vi "Get Keys.vi"(8 "error in":errorcluster, 11 "Object Entry in":refnum<class "Section.lvclass">) -> (0 "error out":errorcluster, 2 "Keys":refnum<class "Key Name.lvclass">[](array[class]), 3 "Object Entry out":refnum<class "Section.lvclass">)   [LabVIEW 2019, in "Electronic Datasheet.lvlib" / "Section.lvclass"]
uses:
  Section.lvclass
  Keyname/Key Name.lvclass
  Section.lvclass/Section.ctl
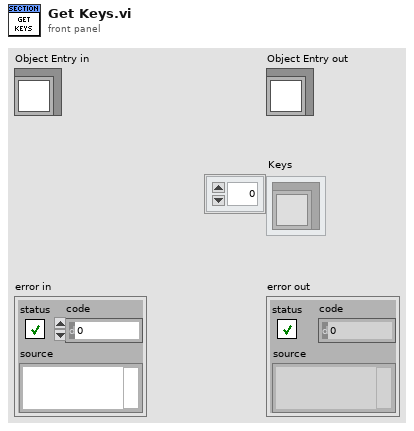
[diagram p1: front panel]
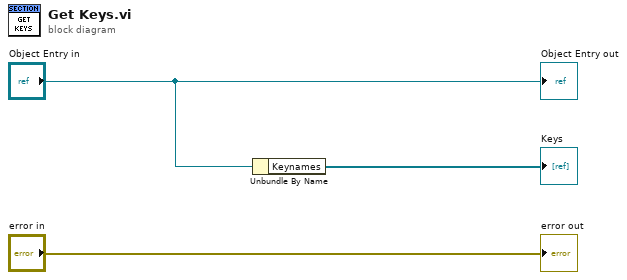
[diagram p0: block diagram]
diagram:
  n1 = Unbundle By Name("Object Entry in") -> ("Keynames"=→"Keys":refnum<class "Key Name.lvclass">[])
  "error out" <- "error in"
  "Object Entry out" <- "Object Entry in"
